vi "FGV Messdaten für logging.vi"(6 "Aktionen":T2, 7 "Temp/Konst.":sgl[](array[numeric]), 8 "error in (no error)":errorcluster caption="Fehler (Eingang, kein Fehler)", 9 "Boolesch":bool, 10 "Aktuelle Zeit":timestamp, 11 "AK Messwerte":T1) -> (0 "error out":errorcluster caption="Fehler (Ausgang)")   [LabVIEW 2020, in "Messdaten.lvlib"]
uses:
  Messdaten.lvlib
  Aktionen FGV Messdaten logging.ctl
  Seiten/FT-IR/FGV FT-IR Gasliste Aktionen.ctl
  Seiten/Log Konfig/Aktionen Trigger.ctl
  Seiten/Log Konfig/Log Sequence FGV Aktion.ctl
  Aktionen FGV Messwerte zusammenfassen.ctl
  Seiten/EL3000/Allgemeine VI/Aktion FGV Werte Standardanalysator.ctl
  Seiten/FT-IR/Algebraic Modul/FGV Algebraic Aktionen.ctl
  Seiten/FT-IR/Aktionen EVID-Codes.ctl
  Gewichtung (Stichprobe).ctl
  Seiten/Log Konfig/LogKonfig.lvlib
  Seiten/FT-IR/TOOLweb Interface Library/TOOLweb Interface Hilfs-VIs.lvlib
  Seiten/FT-IR/FT-IR.lvlib
  Seiten/EL3000/Allgemeine VI/Allgemeine VI.lvlib
  Seiten/FT-IR/Algebraic Modul/Algebraic Modul.lvlib
  Linearisierung V2/Linearisierung v2.lvlib
panel:
  out "Aktuelle Messwerte":sgl[](array[numeric])
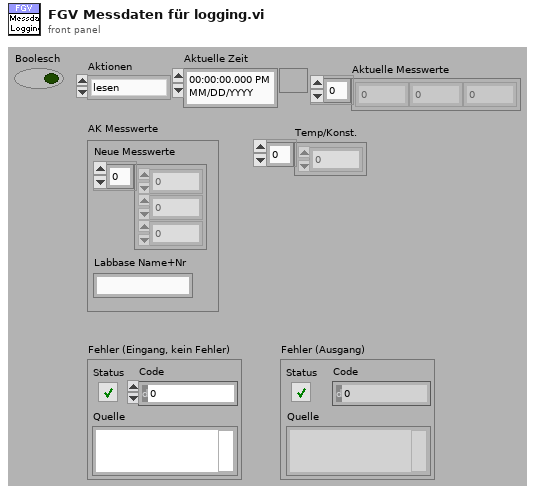
[diagram p1: front panel]
types:
  T1 = cluster{"Neue Messwerte":sgl[], "Labbase Name+Nr":string}
  T2 = typedef "Messdaten.lvlib/Aktionen FGV Messdaten logging.ctl" = enum16{"lesen", "schreiben", "init", "löschen", "werte eintakten", "Flag setzen"}
  T3 = typedef "FT-IR.lvlib/Aktionen EVID-Codes.ctl" = enum16{"lesen", "setzen", "laden", "speichern", "1Hz/5Hz", "Smoothing", "Rolling Average"}
  T4 = typedef "FT-IR.lvlib/Algebraic Modul.lvlib/FGV Algebraic Aktionen.ctl" = enum16{"lesen", "laden", "speichern", "berechnen", "schreiben"}
  T5 = typedef "ABB-EL3000.lvlib/Allgemeine VI.lvlib/Aktion FGV Werte Standardanalysator.ctl" = enum16{"lesen", "FID", "PMA"}
  T6 = typedef "Messdaten.lvlib/Aktionen FGV Messwerte zusammenfassen.ctl" = enum16{"lesen", "FT-IR", "Algebraic", "LabBaseName", "LabBaseNr"}
  T7 = typedef "LogKonfig.lvlib/Log Sequence FGV Aktion.ctl" = enum16{"initialisieren", "lesen", "schreiben", "laden", "speichern", "übertragen"}
  T8 = typedef "LogKonfig.lvlib/Aktionen Trigger.ctl" = enum16{"lesen", "ALLE schreiben", "Trigger prüfen", "Trigger rücksetzen"}
  T9 = typedef "FT-IR.lvlib/FGV FT-IR Gasliste Aktionen.ctl" = enum16{"lesen", "Gasliste FT-IR", "Gasliste ausgelesen", "laden", "speichern", "löschen"}
  T10 = typedef "Messdaten.lvlib/Gewichtung (Stichprobe).ctl" = enum16{"Sample", "Population"}
  T11 = typedef "FT-IR.lvlib/Rolling Average Settings.ctl" = cluster{"Average":u32, "Average via AK:":bool, "Average IAG Software:":bool}
  T12 = typedef "FT-IR.lvlib/1Hz-5Hz Geraet.ctl" = u16
  T13 = typedef "String - Ausgabefeld.ctl" = string
  T14 = cluster{"Index Array":i32[], "Namen Array":string[], "Spektrum File Name":bool}
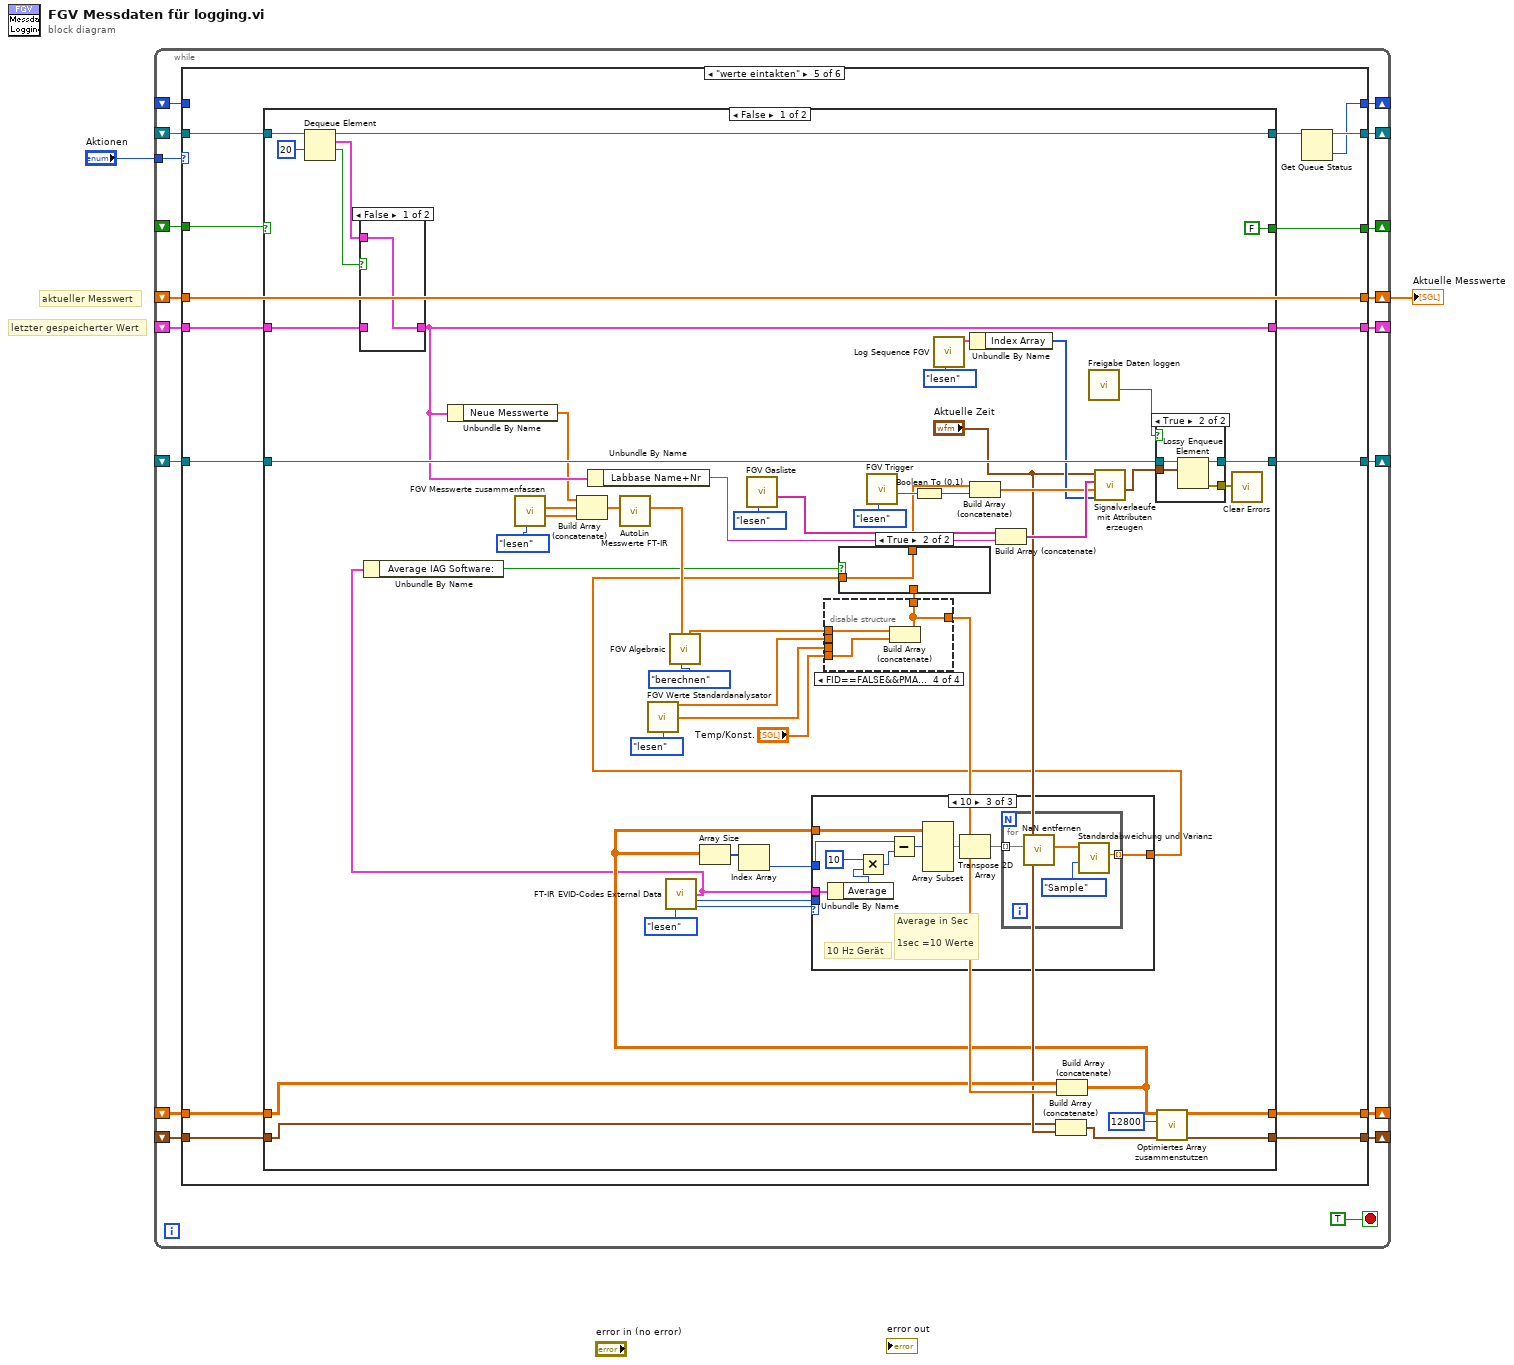
[diagram p0: block diagram]
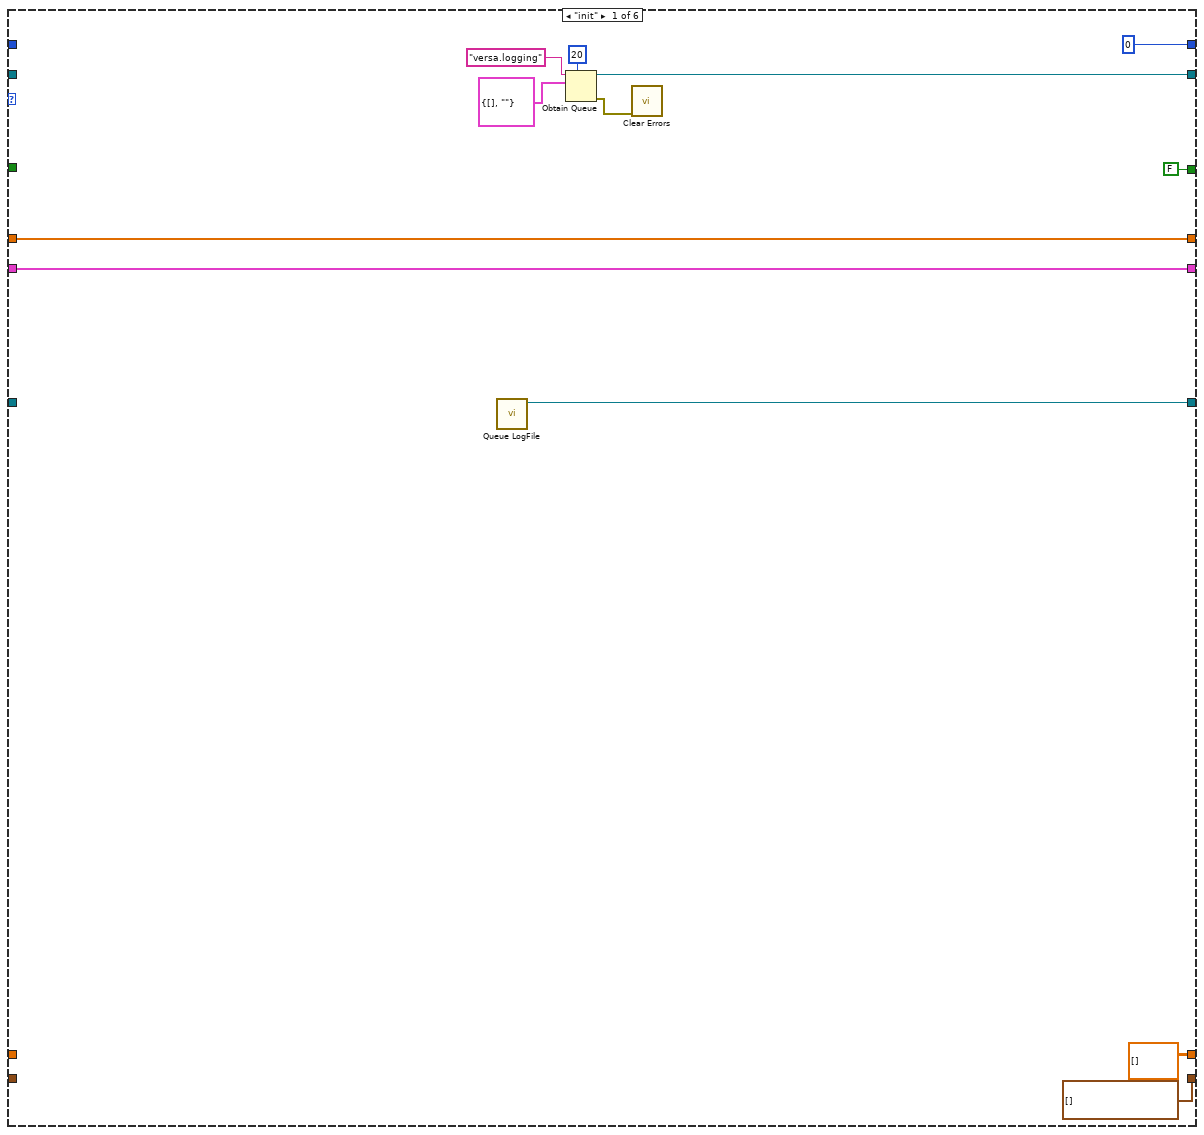
[diagram p2: hidden frame]
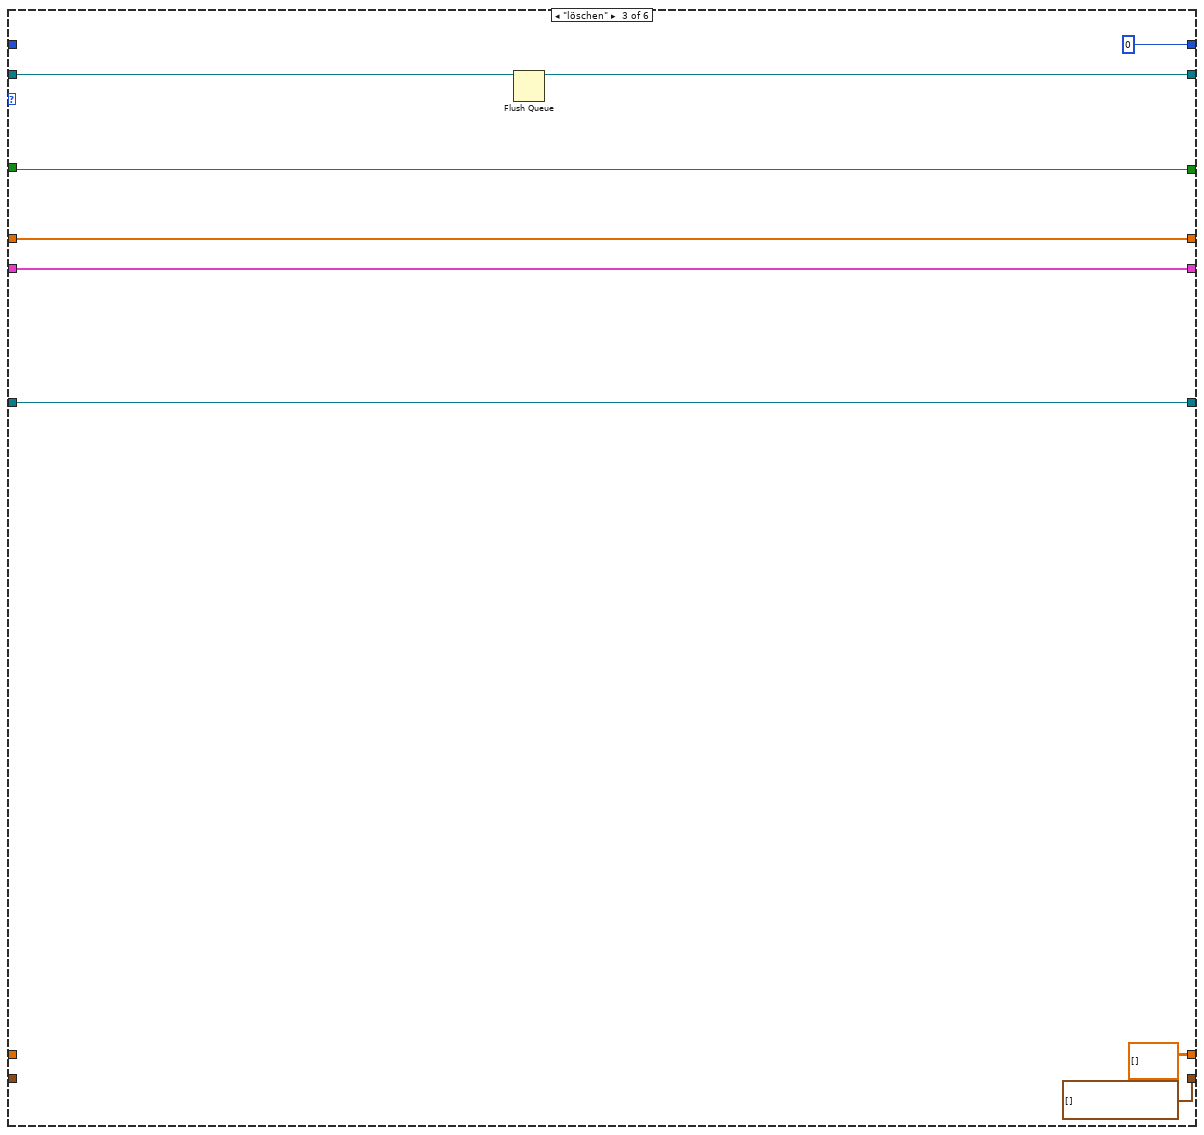
[diagram p4: hidden frame]
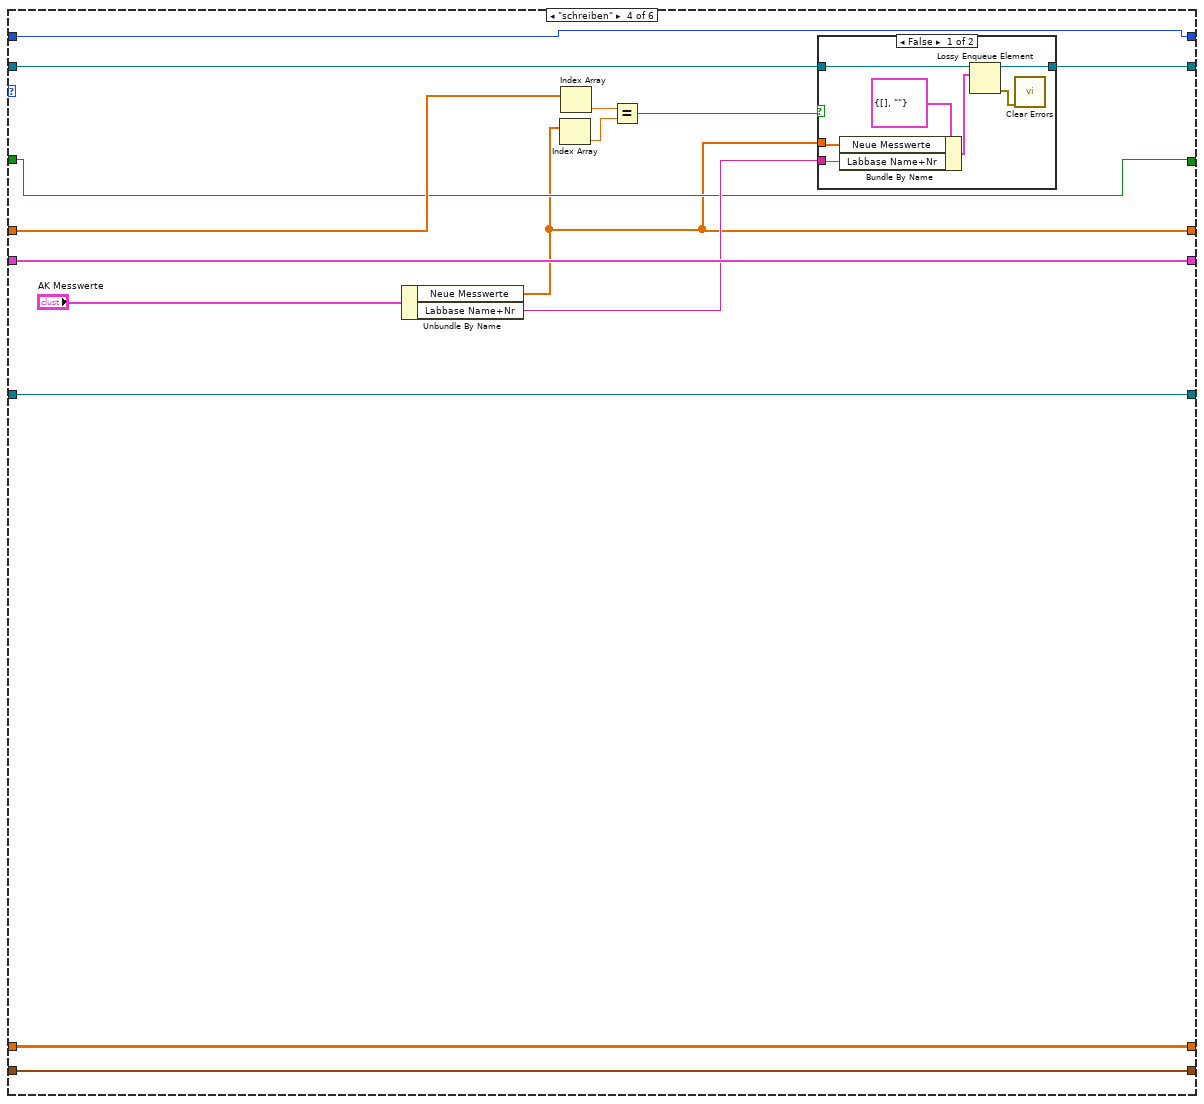
[diagram p5: hidden frame]
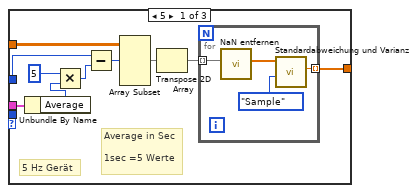
[diagram p8: hidden frame]
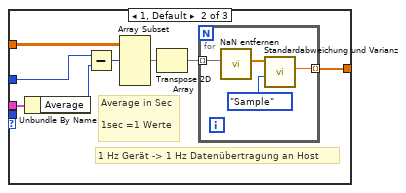
[diagram p9: hidden frame]
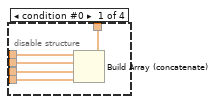
[diagram p10: hidden frame]
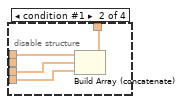
[diagram p11: hidden frame]
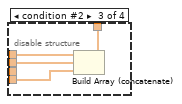
[diagram p12: hidden frame]
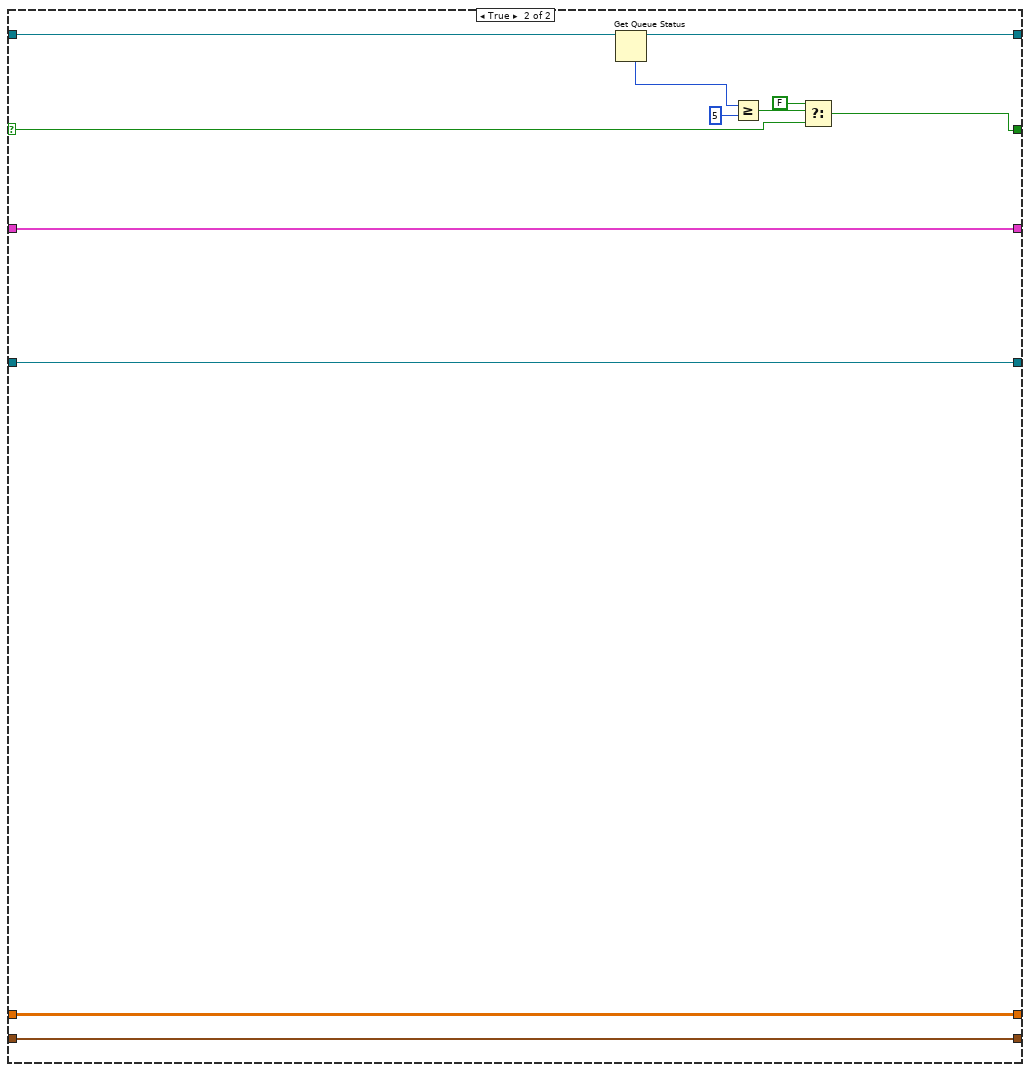
[diagram p15: hidden frame]
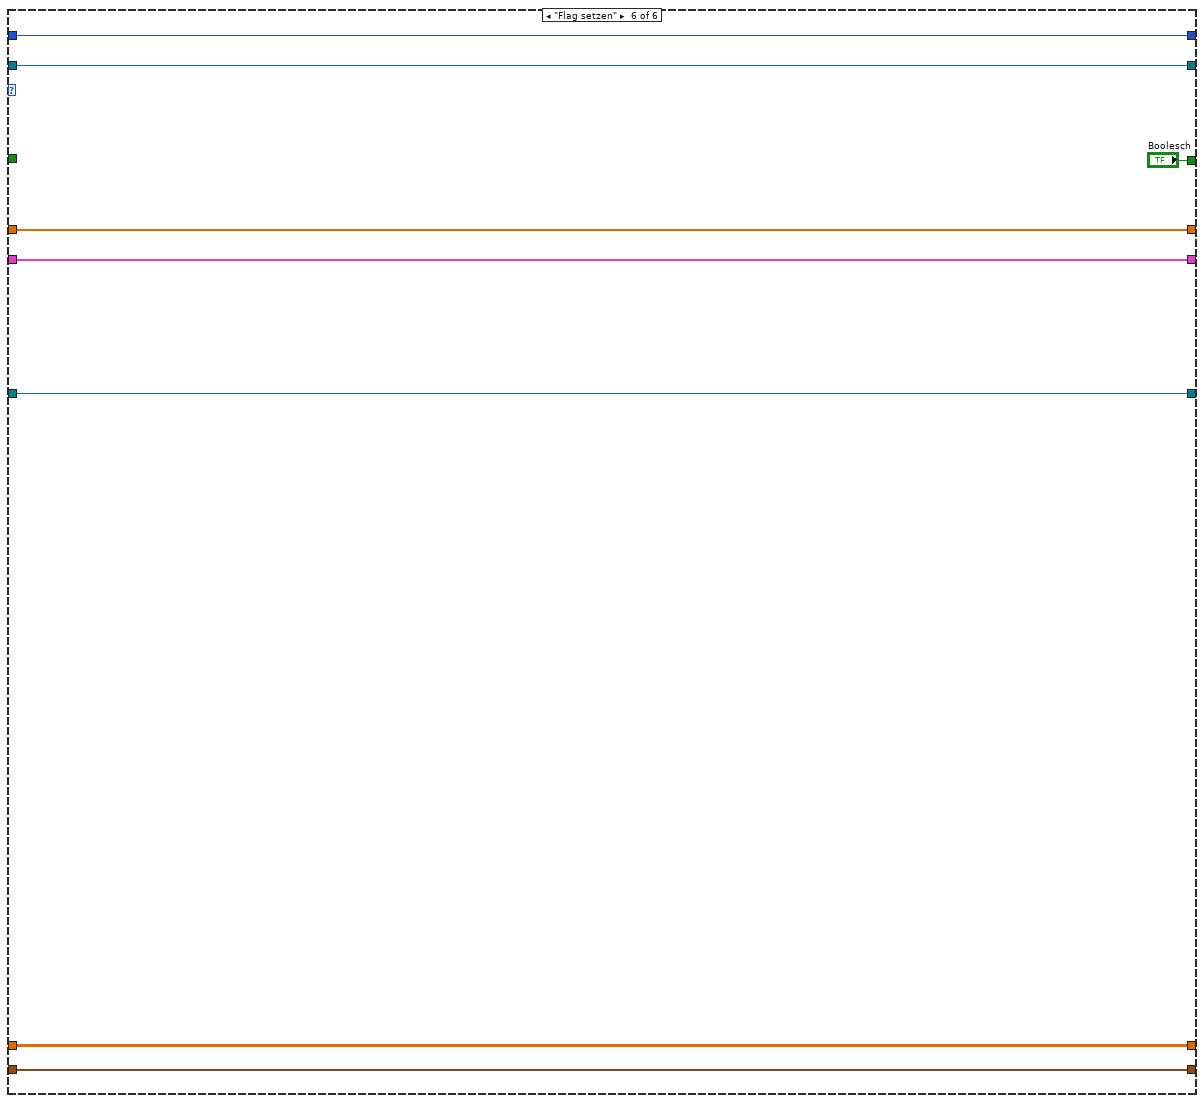
[diagram p16: hidden frame]
diagram:
  # "letzter gespeicherter Wert"
  # "aktueller Messwert"
  n1 = while {
    tunnel: "Aktionen" -> [w19]
    shift-right: [w18] -> w1
    shift-left: _ -> [w17]
    shift-right: [w16] -> _
    shift-left: _ -> [w15]
    shift-right: [w14] -> _
    shift-left: _ -> [w13]
    shift-right: [w12] -> _
    shift-left: _ -> [w11]
    shift-right: [w10] -> _
    shift-left: _ -> [w9]
    shift-right: [w7] -> _
    shift-left: _ -> [w8]
    shift-right: [w6] -> _
    shift-left: _ -> [w5]
    shift-right: [w4] -> _
    shift-left: _ -> [w3]
    stop <- TRUE stop-if-true
    n2 = case shown="\"werte eintakten\"" w19 {
      tunnel: [w32 w40 w49 w52 w87 w223] -> w18
      tunnel: w17 -> [w32 w40 w49 w61 w87 w223]
      tunnel: [w29 w39 w47 w64 w80 w224] -> w16
      tunnel: w15 -> [_ w39 w48 w55 w86 w224]
      tunnel: [w27 w38 w46 w59 w83 w222] -> w14
      tunnel: w13 -> [_ w38 w46 w59 w84 w222]
      tunnel: [w26 w37 w45 w58 w81 w227] -> w12
      tunnel: w11 -> [w26 w37 w45 w58 w82 w227]
      tunnel: [0 ("# elements in queue") w36 0 ("# elements in queue") w54 w79 w225] -> w10
      tunnel: w9 -> [_ w36 _ w54 _ w225]
      tunnel: w8 -> [_ w35 w43 w53 w78 _]
      tunnel: [FALSE ("Boolesch") w35 w43 w53 w77 "Boolesch"] -> w7
      tunnel: [sgl[][] [] ("Messdaten") w34 sgl[][] [] ("Messdaten") w51 w76 w220] -> w6
      tunnel: w5 -> [_ w34 _ w51 w75 w220]
      tunnel: [timestamp[] [] ("Zeitstempeln") w33 timestamp[] [] ("Zeitstempeln") w50 w74 w221] -> w4
      tunnel: w3 -> [_ w33 _ w50 w73 w221]
      frame "init" {
        n3 = call "Queue LogFile.vi"() -> ("Queue (Ausgang)"=w27:refnum<queue>)  [unwired: 6 in, 1 out]
        n4 = Obtain Queue(max queue size (-1, unlimited)=20 ("Maximale Queue-Größe (-1, unbegrenzt)"), name (unnamed)="versa.logging" ("Name (unbenannt)"), element data type=T1 {"Neue Messwerte"=[], "Labbase Name+Nr"=""} ("AK Messwerte")) -> (queue out=w29:refnum<queue>, error out=w28:errorcluster)  [unwired: 2 in, 1 out]
        n5 = call <vilib>:"Clear Errors.vi"("error in (no error)"=w28) -> ()  [unwired: 5 in, 2 out]
      }
      frame "lesen", Default {
      }
      frame "löschen" {
        n6 = Flush Queue(queue=w48) -> (queue out=w47:refnum<queue>)  [unwired: 1 in, 2 out]
      }
      frame "schreiben" {
        n7 = Unbundle By Name("AK Messwerte") -> ("Neue Messwerte"=w52:sgl[], "Labbase Name+Nr"=w57:string)
        n8 = Index Array(array=w52) -> (element=w63:sgl)  [unwired: 1 in]
        n9 = Index Array(array=w61) -> (element=w60:sgl)  [unwired: 1 in]
        n10 = Equal?(x=w60, y=w63) -> (x = y?=w62:bool)
        n11 = case shown="False" w62 {
          tunnel: w55 -> [w71 w72]
          tunnel: [w70 w72] -> w64
          tunnel: w52 -> [w67 _]
          tunnel: w57 -> [w66 _]
          frame False {
            n12 = Bundle By Name(cluster=T1 {"Neue Messwerte"=[], "Labbase Name+Nr"=""} ("AK Messdaten"), "Neue Messwerte"=w67, "Labbase Name+Nr"=w66) -> (w68:T1)
            n13 = Lossy Enqueue Element(queue=w71, element=w68) -> (queue out=w70:refnum<queue>, error out=w69:errorcluster)  [unwired: 1 in, 2 out]
            n14 = call <vilib>:"Clear Errors.vi"("error in (no error)"=w69) -> ()  [unwired: 5 in, 2 out]
          }
          frame True {
          }
        }
      }
      frame "werte eintakten" {
        n15 = case shown="False" w78 {
          selector: w78 -> [_ w212]
          tunnel: w86 -> [w142 w219]
          tunnel: [w141 w218] -> w85
          tunnel: w84 -> [w139 w216]
          tunnel: [w138 w216] -> w83
          tunnel: w82 -> [w126 w217]
          tunnel: [w123 w217] -> w81
          tunnel: [FALSE w210] -> w77
          tunnel: [w104 w209] -> w76
          tunnel: w75 -> [w103 w209]
          tunnel: [w100 w208] -> w74
          tunnel: w73 -> [w99 w208]
          frame False {
            n16 = Dequeue Element(queue=w142, timeout in ms (-1)=20 ("Timeout in ms (-1)")) -> (queue out=w141:refnum<queue>, element=w127:T1, timed out?=w128:bool)  [unwired: 1 in, 1 out]
            n17 = case shown="False" w128 {
              tunnel: w127 -> [w201 _]
              tunnel: [w201 w202] -> w123
              tunnel: w126 -> [_ w202]
              frame False {
              }
              frame True {
              }
            }
            n18 = Unbundle By Name(w123) -> ("Neue Messwerte"=w111:sgl[])
            n19 = call "FGV Messwerte zusammenfassen.vi"("Aktionen"=Aktionen_FGV_Messwerte_zusammenfassen."lesen") -> ("FTIR Status"=w116:sgl[], "Algebraic"=w115:sgl[])  [unwired: 6 in, 3 out]
            n20 = Build Array (concatenate)(w111, w115, w116) -> (w117:sgl[])
            n21 = Unbundle By Name(w123) -> ("Labbase Name+Nr"=w124:string)
            n22 = call "AutoLin Messwerte FT-IR.vi"("FT-IR Rohwerte"=w117) -> ("FT-IR Linearisiert"=w118:sgl[])  [unwired: 10 in]
            n23 = call "FGV Werte Standardanalysator.vi"("Aktion"=Aktion_FGV_Werte_Standardanalysator."lesen") -> ("FID"=w109:sgl[], "PMA"=w108:sgl[])  [unwired: 8 in, 5 out]
            n24 = call "FT-IR EVID-Codes External Data.vi"("Aktionen"=Aktionen_EVID-Codes."lesen") -> ("Rolling Average Settings"=w92:T11, "1Hz/5Hz Leitsystem"=w96:T12, "1Hz/5Hz Gerät"=w97:T12)  [unwired: 9 in, 3 out]
            n25 = Unbundle By Name(w92) -> ("Average IAG Software:"=w89:bool)
            n26 = call "FGV Algebraic.vi"("Aktionen Algebraic"=FGV_Algebraic_Aktionen."berechnen", "Istwerte"=w118) -> ("Messdaten"=w110:sgl[])  [unwired: 5 in, 4 out]
            n27 = call "FGV Gasliste.vi"("Aktionen"=FGV_FT-IR_Gasliste_Aktionen."lesen") -> ("Aktuelle Gasliste gesamt"=w134:T13[])  [unwired: 8 in, 2 out]
            n28 = disable-structure shown="FID==FALSE&&PMA==FALSE, Standard" {
              disable-tunnel: [w189 w193 w197 w198] -> w91
              disable-tunnel: w110 -> [w188 w192 w196 w200]
              disable-tunnel: w109 -> [w187 _ w195 _]
              disable-tunnel: w108 -> [w186 w191 _ _]
              disable-tunnel: "Temp/Konst." -> [w185 w190 w194 w199]
              disable-tunnel: [_ _ _ w198] -> w105
              frame condition #0 {
                n29 = Build Array (concatenate)(w188, w187, w186, w185) -> (w189:sgl[])
              }
              frame condition #1 {
                n30 = Build Array (concatenate)(w192, w191, w190) -> (w193:sgl[])
              }
              frame condition #2 {
                n31 = Build Array (concatenate)(w196, w195, w194) -> (w197:sgl[])
              }
              frame condition #3 (active) {
                n32 = Build Array (concatenate)(w200, w199) -> (w198:sgl[])
              }
            }
            n33 = call "FGV Trigger.vi"("Aktion"=Aktionen_Trigger."lesen") -> ("Trigger gesetzt?"=w135:bool)  [unwired: 7 in, 3 out]
            n34 = Boolean To (0,1)(Boolean=w135) -> (0, 1=w136:i16)
            n35 = call "Log Sequence FGV.vi"("Aktion"=Log_Sequence_FGV_Aktion."lesen") -> ("Cluster (out)"=w121:T14)  [unwired: 10 in]
            n36 = Unbundle By Name(w121) -> ("Index Array"=w120:i32[])
            n37 = Build Array (concatenate)(w134, w124) -> (w131:T13[])
            n38 = Build Array (concatenate)(w99, "Aktuelle Zeit") -> (w101:timestamp[])
            n39 = Build Array (concatenate)(w103, w105) -> (w95:sgl[][])
            n40 = Array Size(array=w95) -> (size(s)=w94:i32[])
            n41 = Index Array(array=w94) -> (element=w93:i32)  [unwired: 1 in]
            n42 = case shown="10" w97 {
              tunnel: w96 -> [_ _ _]
              tunnel: w95 -> [w154 w166 w180]
              tunnel: w93 -> [w153 w165 w179]
              tunnel: [w152 w164 w178] -> w88
              tunnel: w92 -> [w148 w160 w174]
              frame 5 {
                # "Average in Sec\n\n1sec =5 Werte"
                # "5 Hz Gerät"
                n43 = Unbundle By Name(w148) -> ("Average"=w146:u32)
                n44 = Multiply(x=5 ("y"), y=w146) -> (x*y=w145:u32)
                n45 = Subtract(x=w153, y=w145) -> (x-y=w151:u32)
                n46 = Array Subset(array=w154, index (row)=w151) -> (w150:sgl[][])  [unwired: 3 in]
                n47 = Transpose 2D Array(2D array=w150) -> (transposed array=w149:sgl[][])
                n48 = for {
                  tunnel: w149 -> [w155] mode=indexing
                  tunnel: [w157] -> w152 mode=indexing
                  n49 = call "NaN entfernen.vi"("Messdaten"=w155) -> ("Messdaten"=w156:sgl[])  [unwired: 10 in]
                  n50 = call "Standardabweichung und Varianz.vi"("Gewichtung (Stichprobe)"=Gewichtung_(Stichprobe)."Sample", "X"=w156) -> ("Mittelwert"=w157:sgl)  [unwired: 7 in, 2 out]
                }
              }
              frame 1, Default {
                # "1 Hz Gerät -> 1 Hz Datenübertragung an Host"
                # "Average in Sec\n\n1sec =1 Werte"
                n51 = Unbundle By Name(w160) -> ("Average"=w159:u32)
                n52 = Subtract(x=w165, y=w159) -> (x-y=w163:u32)
                n53 = Array Subset(array=w166, index (row)=w163) -> (w162:sgl[][])  [unwired: 3 in]
                n54 = Transpose 2D Array(2D array=w162) -> (transposed array=w161:sgl[][])
                n55 = for {
                  tunnel: w161 -> [w167] mode=indexing
                  tunnel: [w169] -> w164 mode=indexing
                  n56 = call "NaN entfernen.vi"("Messdaten"=w167) -> ("Messdaten"=w168:sgl[])  [unwired: 10 in]
                  n57 = call "Standardabweichung und Varianz.vi"("Gewichtung (Stichprobe)"=Gewichtung_(Stichprobe)."Sample", "X"=w168) -> ("Mittelwert"=w169:sgl)  [unwired: 7 in, 2 out]
                }
              }
              frame 10 {
                # "10 Hz Gerät"
                # "Average in Sec\n\n1sec =10 Werte"
                n58 = Unbundle By Name(w174) -> ("Average"=w172:u32)
                n59 = Multiply(x=10 ("y"), y=w172) -> (x*y=w171:u32)
                n60 = Subtract(x=w179, y=w171) -> (x-y=w177:u32)
                n61 = Array Subset(array=w180, index (row)=w177) -> (w176:sgl[][])  [unwired: 3 in]
                n62 = Transpose 2D Array(2D array=w176) -> (transposed array=w175:sgl[][])
                n63 = for {
                  tunnel: w175 -> [w181] mode=indexing
                  tunnel: [w183] -> w178 mode=indexing
                  n64 = call "NaN entfernen.vi"("Messdaten"=w181) -> ("Messdaten"=w182:sgl[])  [unwired: 10 in]
                  n65 = call "Standardabweichung und Varianz.vi"("Gewichtung (Stichprobe)"=Gewichtung_(Stichprobe)."Sample", "X"=w182) -> ("Mittelwert"=w183:sgl)  [unwired: 7 in, 2 out]
                }
              }
            }
            n66 = case shown="True" w89 {
              tunnel: w91 -> [w143 _]
              tunnel: [w143 w144] -> w90
              tunnel: w88 -> [_ w144]
              frame False {
              }
              frame True {
              }
            }
            n67 = Build Array (concatenate)(w90, w136) -> (w130:sgl[])
            n68 = call "Freigabe Daten loggen.vi"() -> ("Daten loggen"=w140:bool)  [unwired: 11 in]
            n69 = call "Signalverlaeufe mit Attributen erzeugen.vi"("Log Sequence"=w120, "Messwerte"=w130, "Namen"=w131, "Zeitstempel"="Aktuelle Zeit") -> ("Signalverläufe"=w137:waveform(dbl)[])  [unwired: 7 in]
            n70 = case shown="True" w140 {
              tunnel: w139 -> [w203 w207]
              tunnel: [w203 w206] -> w138
              tunnel: [_ w205] -> w125
              tunnel: w137 -> [_ w204]
              frame False {
              }
              frame True {
                n71 = Lossy Enqueue Element(queue=w207, element=w204) -> (queue out=w206:refnum<queue>, error out=w205:errorcluster)  [unwired: 1 in, 2 out]
              }
            }
            n72 = call "Optimiertes Array zusammenstutzen.vi"("Zeitstempeln"=w101, "Anzahl Elemente"=12800, "Messdaten"=w95) -> ("Zeitstempeln"=w100:timestamp[], "Messdaten"=w104:sgl[][])  [unwired: 7 in]
            n73 = call <vilib>:"Clear Errors.vi"("error in (no error)"=w125) -> ()  [unwired: 5 in, 2 out]
          }
          frame True {
            n74 = Get Queue Status(queue=w219) -> (queue out=w218:refnum<queue>, # elements in queue=w215:i32)  [unwired: 2 in, 6 out]
            n75 = Greater Or Equal?(x=w215, y=5) -> (x >= y?=w213:bool)
            n76 = Select(t=FALSE, s=w213, f=w212) -> (s? t:f=w210:bool)
          }
        }
        n77 = Get Queue Status(queue=w85) -> (queue out=w80:refnum<queue>, # elements in queue=w79:i32)  [unwired: 2 in, 6 out]
      }
      frame "Flag setzen" {
      }
    }
  }
  "Aktuelle Messwerte" <- w1
